vi "Build Sources Map.vi"() -> (2 "Sources":T1(c390))   [LabVIEW 2020, in "VolatusGUI.lvlib" / "BluelinesRedlines Source.lvclass"]
uses:
  BluelinesRedlines Source.lvclass
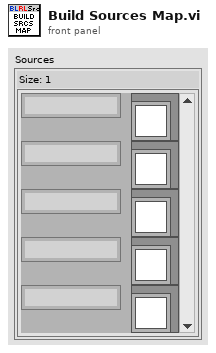
[diagram p1: front panel]
types:
  T1 = map{string, refnum<class "BluelinesRedlines Source.lvclass">}
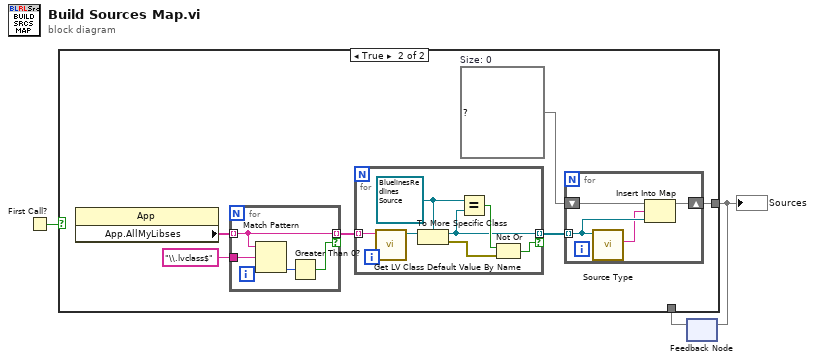
[diagram p0: block diagram]
diagram:
  n1 = First Call?() -> (First Call?: T/F=w1:bool)
  n2 = feedback #1() -> (w2:T1)  [unwired: 1 in]
  n3 = case shown="True" w1 {
    tunnel: [w4 w5] -> w3
    tunnel: w2 -> [w4 _]
    frame False {
    }
    frame True {
      w6 = T1 {}  # Size: 0
      n4 = property class="App"() -> ("App.AllMyLibses"=w10:string[])  [unwired: 2 in, 2 out]
      n5 = for {
        tunnel: w10 -> [w23] mode=indexing
        tunnel: "\\.lvclass$" -> [w25]
        tunnel: [w23] -> w8 mode=indexing if=w22
        n6 = Match Pattern(string=w23, regular expression=w25) -> (offset past match=w24:i32)  [unwired: 1 in, 3 out]
        n7 = Greater Than 0?(x=w24) -> (x > 0?=w22:bool)
      }
      n8 = for {
        tunnel: w8 -> [w21] mode=indexing
        tunnel: [w16] -> w7 mode=indexing if=w15
        w19 = refnum<class "BluelinesRedlines Source.lvclass"> refnum ("VolatusGUI:BluelinesRedlines Source.lvclass")
        n9 = call <vilib>:"Get LV Class Default Value By Name.vi"("class name"=w21) -> ("object"=w20:refnum<class>)  [unwired: 9 in, 1 out]
        n10 = To More Specific Class(target class=w19, reference=w20) -> (specific class reference=w16:refnum<class "BluelinesRedlines Source.lvclass">, error out=w18:errorcluster)  [unwired: 1 in]
        n11 = Equal?(x=w19, y=w16) -> (x = y?=w17:bool)
        n12 = Not Or(1:w18, 2:w17) -> (0:w15:bool)
      }
      n13 = for {
        tunnel: w7 -> [w13] mode=indexing
        shift-right: [w11] -> w5
        shift-left: w6 -> [w14]
        n14 = call-dynamic "Source Type.vi"("BluelinesRedlines Source in"=w13) -> ("Source Type"=w12:string)  [unwired: 10 in]
        n15 = Insert Into Map(map in=w14, key=w12, value=w13) -> (map out=w11:T1)  [unwired: 2 out]
      }
    }
  }
  "Sources" <- w3
  n16 = feedback-in #1(w3) -> ()
